vi "Save data.vi"(8 "error in (no error)":errorcluster, 10 "signal out":waveform(dbl), 11 "Logging Txt in":refnum<class "Logging Txt.lvclass">) -> (0 "error out":errorcluster, 3 "Logging Txt out":refnum<class "Logging Txt.lvclass">)   [LabVIEW 2020, in "Logging Txt.lvlib" / "Logging Txt.lvclass"]
uses:
  Logging Txt.lvclass
  Logging Txt.lvclass/Logging Txt.ctl
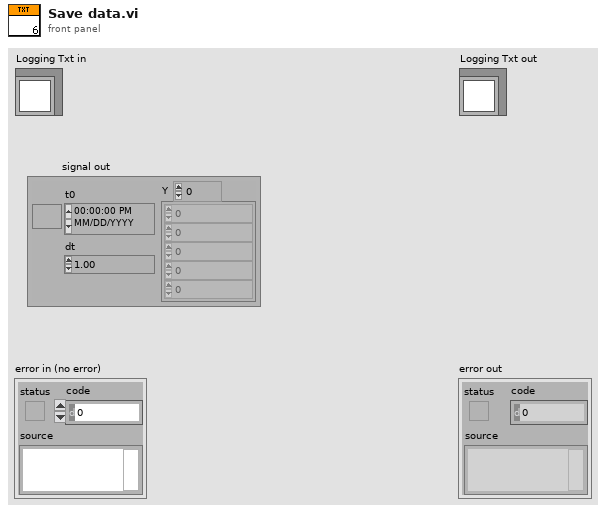
[diagram p1: front panel]
types:
  T1 = enum16{"open", "replace", "create", "open or create", "replace or create", "replace or create with confirmation"}
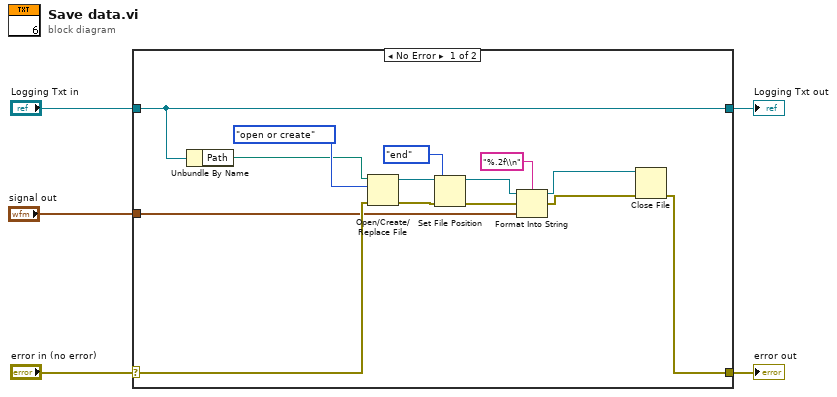
[diagram p0: block diagram]
diagram:
  n1 = case shown="No Error" "error in (no error)" {
    selector: "error in (no error)" -> [w8 w21]
    tunnel: [w7 w21] -> w4
    tunnel: [w19 w20] -> w2
    tunnel: "Logging Txt in" -> [w19 w20]
    tunnel: "signal out" -> [w6 _]
    frame No Error {
      n2 = Unbundle By Name(w19) -> ("Path"=w9:path)
      n3 = Open/Create/Replace File(file path (use dialog)=w9, error in=w8, operation (0:open)=T1."open or create") -> (refnum out=w17:refnum<file>, error out=w16:errorcluster)  [unwired: 3 in, 1 out]
      n4 = Set File Position(refnum=w17, from (0:start)=enum16{"start", "end", "current"}."end", error in=w16) -> (refnum out=w14:refnum<file>, error out=w13:errorcluster)  [unwired: 1 in]
      n5 = Format Into String(format string="%.2f\\n", initial string=w14, error in=w13, w6) -> (resulting string=w11:refnum<file>, error out=w12:errorcluster)
      n6 = Close File(refnum=w11, error in=w12) -> (error out=w7:errorcluster)  [unwired: 1 out]
    }
    frame Error {
    }
  }
  "error out" <- w4
  "Logging Txt out" <- w2
